vi "PH_HamamatsuCamera.ProcCases.vi"(0 "i ref in":refnum<vi>, 1 "selector":string, 2 "data":T1, 3 "call cluster":T2={"Object"="", "Selector"="", "CallType"=enum."synchronous", "Async Object"="", "Async Selector"="", "Data Descriptor"="", "Data"=[], "Error #"=0, "Expire"=0}, 5 "error in":errorcluster) -> (14 "i ref out":refnum<vi>, 17 "answer cluster":T2={"Object"="", "Selector"="", "CallType"=enum."synchronous", "Async Object"="", "Async Selector"="", "Data Descriptor"="", "Data"=[], "Error #"=0, "Expire"=0}, 19 "error out":errorcluster)   [LabVIEW 2014, in "PH_HamamatsuCamera.lvlib"]
doc: "This method is called by a process from within the default case in the event loop. The methods of a class that are linked to events will be called from THIS method. Add your code here."
uses:
  PH_HamamatsuCamera.lvlib
  CS_Core/CSSystem/CoreDefs/CoreDefs.call_type.ctl
  CS_Core/BaseProcess/BaseProcess.descriptor string definition.ctl
  CS_Core/CSSystem/CoreDefs/CoreDefs.rawDataType.ctl
  PH_HamamatsuCamera.Trigger Parameter.ctl
  PH_HamamatsuCamera.ROI.ctl
  CS_Core/CSSystem/CoreLib/CoreLib.string 2 byte array.vi
  CS_Core/CSSystem/CoreLib/CoreLib.byte array 2 double.vi
  CS_Core/CSSystem/CoreLib/CoreLib.byte array 2 string.vi
  CS_Core/CSSystem/CoreLib/CoreLib.byte array 2 int.vi
  CS_Core/CSSystem/CoreLib/CoreLib.lvlib
  CS_Core/BaseProcess/BaseProcess.lvlib
  CS_Core/CAEObj/CAEObj.lvlib
  PH_Basics/PH_PSDBWriter/PH_PSDBWriter.lvlib
  PH_Basics/PH_Cam_BaseClass/PH_Cam_BaseClass.lvlib
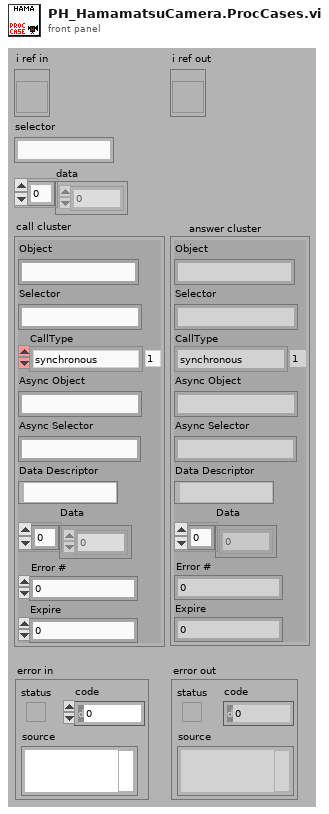
[diagram p1: front panel]
types:
  T1 = typedef "CoreDefs.rawDataType.ctl" = i8[]
  T2 = typedef "CoreDefs.call_type.ctl" = cluster{"Object":string, "Selector":string, "CallType":enum16{"simple", "synchronous", "asynchronous"}, "Async Object":string, "Async Selector":string, "Data Descriptor":T3, "Data":T1, "Error #":i32, "Expire":u32}
  T3 = typedef "BaseProcess.lvlib/BaseProcess.descriptor string definition.ctl" = string
  T4 = typedef "PH_HamamatsuCamera.lvlib/PH_HamamatsuCamera.Trigger Parameter.ctl" = cluster{"Mode":u32, "Polarity":u32, "Times":u32, "Delay":dbl}
  T5 = typedef "PH_HamamatsuCamera.lvlib/PH_HamamatsuCamera.ROI.ctl" = cluster{"Horizontal Offset":i32, "Vertical Offset":i32, "Horizontal Width":i32, "Vertical Width":i32}
  T6 = typedef "PH_PSDBWriter.lvlib/PH_PSDBWriter.PHELIX-Subsystems.ctl" = i32
  T7 = typedef "PH_HamamatsuCamera.lvlib/PH_HamamatsuCamera.i attribute.ctl" = cluster{"Gui Refs":cluster{"Camera Details":refnum<vi>, "ROI":refnum<vi>, "Set ROI to Maximum":refnum<vi>, "Trigger Parameters":refnum<vi>, "Brightness":refnum<vi>, "Shutter":refnum<vi>, "Gain":refnum<vi>, "Trigger Timeout":refnum<vi>, "Trigger Polarity":refnum<vi>, "Trigger Mode":refnum<vi>, "Parameters":refnum<vi>, "Set Cam Parameter":refnum<vi>, "Parameter to set":refnum<vi>, "Value to set":refnum<vi>}, "Cam":cluster{"Handle":i32, "Details":cluster{"Model":string, "Camera ID":string, "Firmware":string}, "Buffer Info":cluster{"height":u32, "width":u32, "datatype":u32}}, "H Offset":cluster{"Value":i32, "Minimum":i32, "Maximum":i32, "Increment":i32}, "V Offset":cluster{"Value":i32, "Minimum":i32, "Maximum":i32, "Increment":i32}, "H Width":cluster{"Value":i32, "Minimum":i32, "Maximum":i32, "Increment":i32}, "V Width":cluster{"Value":i32, "Minimum":i32, "Maximum":i32, "Increment":i32}, "Trigger Parameters":T4, "Trigger Timeout":u32, "Parameters":T8[], "Indicees Cam Parameters":cluster{"Brightness":i32, "Shutter":i32, "Gain":i32}, "Wanted Values":cluster{"Trigger Settings":T4[], "ROI":T5[], "Parameter":cluster{"Name":string, "Value":dbl}[]}}
  T8 = typedef "PH_HamamatsuCamera.lvlib/PH_HamamatsuCamera.Parameter Set.ctl" = cluster{"Parameter":string, "Value":dbl, "Writable":bool, "Range":cluster{"min":dbl, "max":dbl, "step":dbl}, "Default":dbl, "Value Names":cluster{"Name":string, "Value":dbl}[], "Text Values":bool}
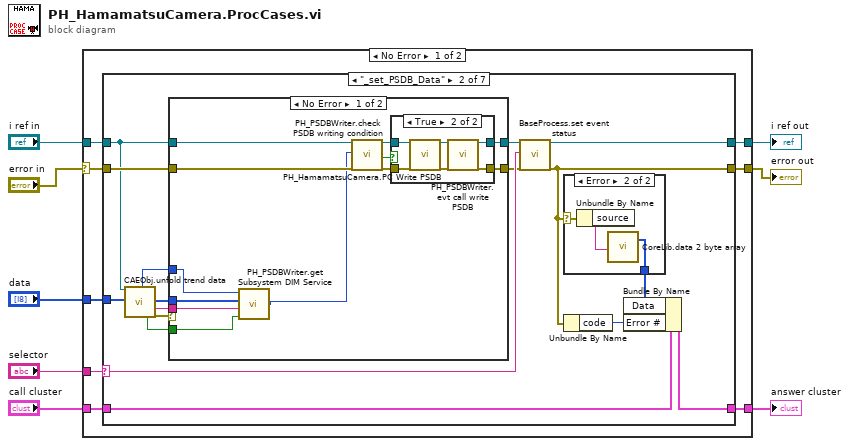
[diagram p0: block diagram]
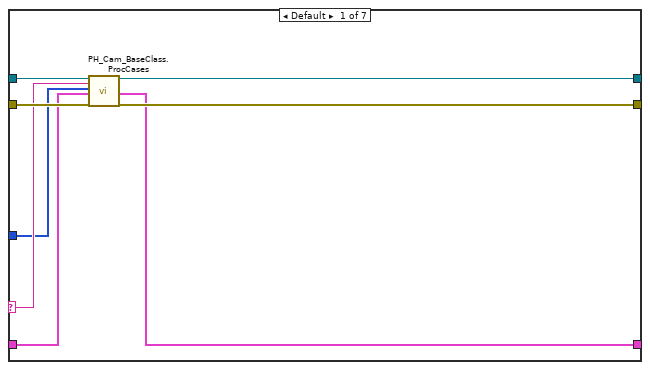
[diagram p2: hidden frame]
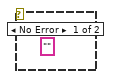
[diagram p5: hidden frame]
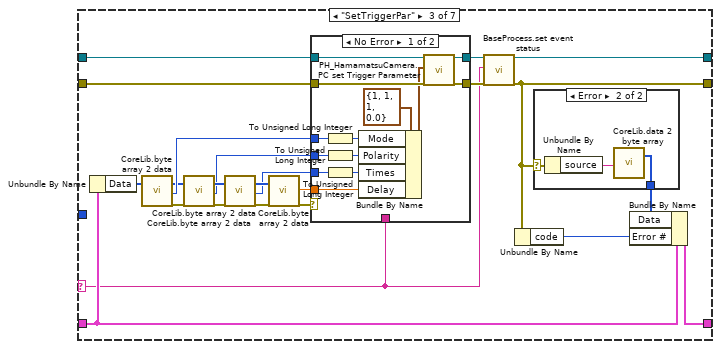
[diagram p6: hidden frame]
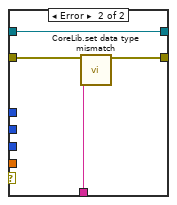
[diagram p8: hidden frame]
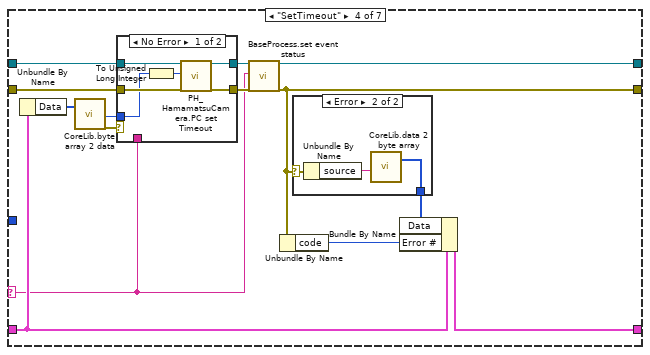
[diagram p9: hidden frame]
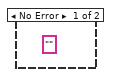
[diagram p10: hidden frame]
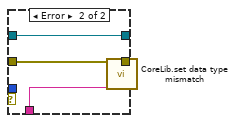
[diagram p11: hidden frame]
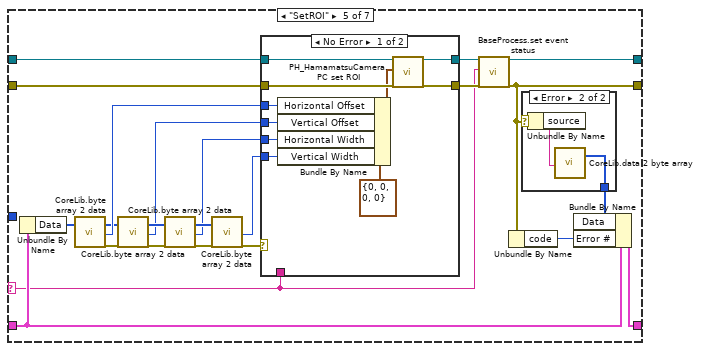
[diagram p12: hidden frame]
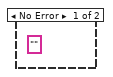
[diagram p13: hidden frame]
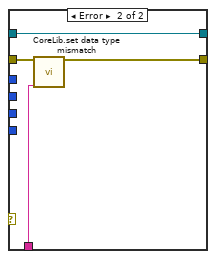
[diagram p14: hidden frame]
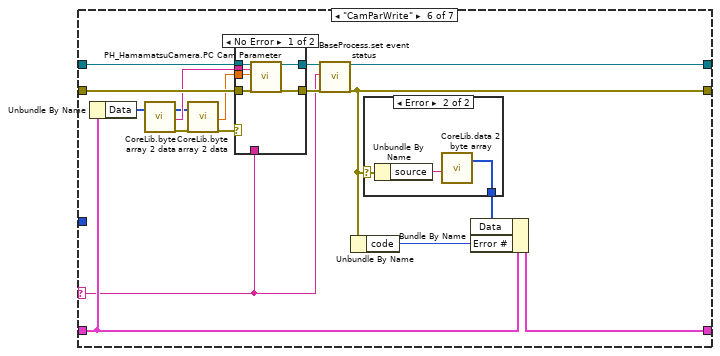
[diagram p15: hidden frame]
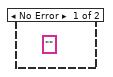
[diagram p16: hidden frame]
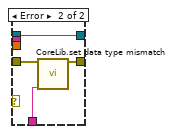
[diagram p17: hidden frame]
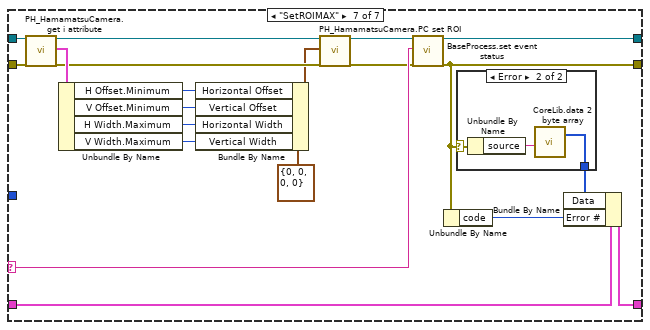
[diagram p18: hidden frame]
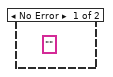
[diagram p19: hidden frame]
diagram:
  n1 = case shown="No Error" "error in" {
    selector: "error in" -> [w9 w231]
    tunnel: "selector" -> [w16 _]
    tunnel: [w15 w230] -> w7
    tunnel: "call cluster" -> [w14 w230]
    tunnel: "i ref in" -> [w13 w232]
    tunnel: [w12 w232] -> w4
    tunnel: [w11 w231] -> w3
    tunnel: "data" -> [w10 _]
    frame No Error {
      n2 = case shown="\"_set_PSDB_Data\"" w16 {
        selector: w16 -> [w19 w37 w81 w115 w151 w185 w220]
        tunnel: w13 -> [w18 w28 w89 w123 w159 w193 w226]
        tunnel: [w24 w36 w80 w114 w150 w184 w219] -> w12
        tunnel: w14 -> [w20 w40 w86 w120 w156 w190 w223]
        tunnel: [w21 w39 w85 w119 w155 w189 w222] -> w15
        tunnel: w9 -> [w23 w29 w88 w122 w158 w192 w225]
        tunnel: [w22 w38 w82 w116 w152 w186 w221] -> w11
        tunnel: w10 -> [w17 w25 _ _ _ _ _]
        frame Default {
          # "In the default case, always call the ProcCase method of the parent class"
          n3 = call "PH_Cam_BaseClass.ProcCases.vi"("i ref in"=w18, "selector"=w19, "data"=w17, "call cluster"=w20, "error in"=w23) -> ("i ref out"=w24:refnum<vi>, "answer cluster"=w21:T2, "error out"=w22:errorcluster)  [unwired: 12 in]
        }
        frame "_set_PSDB_Data" {
          n4 = call "CAEObj.unfold trend data.vi"("i ref in"=w28, "raw trend data"=w25) -> ("quality"=w30:i32, "no link"=w33:bool, "data"=w31:i8[], "typeDescriptor"=w32:string, "error out"=w34:errorcluster)  [unwired: 9 in, 4 out]
          n5 = case shown="No Error" w34 {
            tunnel: w29 -> [w53 w63]
            tunnel: [w52 w62] -> w27
            tunnel: [w51 w63] -> w26
            tunnel: w28 -> [w49 w62]
            tunnel: w33 -> [w43 _]
            tunnel: w32 -> [w44 _]
            tunnel: w31 -> [w46 _]
            tunnel: w30 -> [w45 _]
            frame No Error {
              n6 = call "PH_PSDBWriter.get Subsystem DIM Service.vi"("no link"=w43, "typeDescriptor"=w44, "data"=w46, "quality"=w45) -> ("PHELIX Subsystems"=w42:T6)
              n7 = call "PH_PSDBWriter.check PSDB writing condition.vi"("i ref in"=w49, "wanted Subsystem"=w42, "error IO"=w53) -> ("i ref out"=w48:refnum<vi>, "write PSDB?"=w47:bool, "error out"=w50:errorcluster)  [unwired: 14 in]
              n8 = case shown="True" w47 {
                tunnel: w50 -> [w54 w61]
                tunnel: [w55 w58] -> w52
                tunnel: [w54 w56] -> w51
                tunnel: w48 -> [w55 w60]
                frame False {
                }
                frame True {
                  n9 = call "PH_HamamatsuCamera.PC Write PSDB.vi"("i ref in"=w60, "error IO"=w61) -> ("i ref out"=w59:refnum<vi>, "error out"=w57:errorcluster)  [unwired: 16 in]
                  n10 = call "PH_PSDBWriter.evt call write PSDB.vi"("i ref in"=w59, "error in (no error)"=w57) -> ("i ref out"=w58:refnum<vi>, "error out"=w56:errorcluster)  [unwired: 16 in]
                }
              }
            }
            frame Error {
            }
          }
          n11 = call "BaseProcess.set event status.vi"("i ref in"=w27, "EventStatus"=w37, "error in (no error)"=w26) -> ("i ref out"=w36:refnum<vi>, "error out"=w38:errorcluster)  [unwired: 14 in, 1 out]
          n12 = case shown="Error" w38 {
            selector: w38 -> [_ w66]
            tunnel: [_ w64] -> w35
            frame No Error {
              (unwired) "" ("source")
            }
            frame Error {
              n13 = Unbundle By Name(w66) -> ("source"=w65:string)
              n14 = call-poly "CoreLib.data 2 byte array.vi"("string"=w65) -> ("byteArray out"=w64:T1)  [unwired: 18 in]
            }
          }
          n15 = Unbundle By Name(w38) -> ("code"=w41:i32)
          n16 = Bundle By Name(cluster=w40, "Data"=w35, "Error #"=w41) -> (w39:T2)
        }
        frame "SetTriggerPar" {
          n17 = Unbundle By Name(w86) -> ("Data"=w79:T1)
          n18 = call-poly "CoreLib.byte array 2 data.vi"("byteArray"=w79) -> ("byteArray out"=w72:T1, "i32"=w73:i32, "error out"=w77:errorcluster)  [unwired: 16 in]
          n19 = call-poly "CoreLib.byte array 2 data.vi"("byteArray"=w72, "error in (no error)"=w77) -> ("byteArray out"=w71:T1, "i32"=w69:i32, "error out"=w75:errorcluster)  [unwired: 15 in]
          n20 = call-poly "CoreLib.byte array 2 data.vi"("byteArray"=w71, "error in (no error)"=w75) -> ("byteArray out"=w70:T1, "i32"=w68:i32, "error out"=w76:errorcluster)  [unwired: 15 in]
          n21 = call-poly "CoreLib.byte array 2 data.vi"("byteArray"=w70, "error in (no error)"=w76) -> ("d64"=w67:dbl, "error out"=w74:errorcluster)  [unwired: 15 in, 1 out]
          n22 = case shown="No Error" w74 {
            tunnel: [w94 w109] -> w84
            tunnel: w89 -> [w104 w109]
            tunnel: w88 -> [w105 w108]
            tunnel: [w93 w107] -> w83
            tunnel: w81 -> [_ w106]
            tunnel: w73 -> [w101 _]
            tunnel: w69 -> [w99 _]
            tunnel: w68 -> [w98 _]
            tunnel: w67 -> [w97 _]
            frame No Error {
              n23 = To Unsigned Long Integer(number=w101) -> (unsigned 32bit integer=w100:u32)
              n24 = To Unsigned Long Integer(number=w99) -> (unsigned 32bit integer=w96:u32)
              n25 = To Unsigned Long Integer(number=w98) -> (unsigned 32bit integer=w95:u32)
              n26 = Bundle By Name(cluster=T4 {"Mode"=1, "Polarity"=1, "Times"=1, "Delay"=0.0} ("Trigger Parameters"), "Mode"=w100, "Polarity"=w96, "Times"=w95, "Delay"=w97) -> (w102:T4)
              n27 = call "PH_HamamatsuCamera.PC set Trigger Parameter.vi"("i ref in"=w104, "Trigger Parameters"=w102, "error in (no error)"=w105) -> ("i ref out"=w94:refnum<vi>, "error out"=w93:errorcluster)  [unwired: 15 in]
            }
            frame Error {
              n28 = call "CoreLib.set data type mismatch.vi"("error in (no error)"=w108, "error source"=w106) -> ("error out"=w107:errorcluster)  [unwired: 17 in]
            }
          }
          n29 = call "BaseProcess.set event status.vi"("i ref in"=w84, "EventStatus"=w81, "error in (no error)"=w83) -> ("i ref out"=w80:refnum<vi>, "error out"=w82:errorcluster)  [unwired: 14 in, 1 out]
          n30 = Unbundle By Name(w82) -> ("code"=w87:i32)
          n31 = case shown="Error" w82 {
            selector: w82 -> [_ w92]
            tunnel: [_ w91] -> w78
            frame No Error {
            }
            frame Error {
              n32 = Unbundle By Name(w92) -> ("source"=w90:string)
              n33 = call-poly "CoreLib.data 2 byte array.vi"("string"=w90) -> ("byteArray out"=w91:T1)  [unwired: 18 in]
            }
          }
          n34 = Bundle By Name(cluster=w86, "Data"=w78, "Error #"=w87) -> (w85:T2)
        }
        frame "SetTimeout" {
          n35 = Unbundle By Name(w120) -> ("Data"=w113:T1)
          n36 = call-poly "CoreLib.byte array 2 data.vi"("byteArray"=w113) -> ("i32"=w112:i32, "error out"=w111:errorcluster)  [unwired: 16 in, 1 out]
          n37 = case shown="No Error" w111 {
            tunnel: [w128 w136] -> w118
            tunnel: w123 -> [w131 w136]
            tunnel: w122 -> [w132 w135]
            tunnel: [w127 w134] -> w117
            tunnel: w115 -> [_ w133]
            tunnel: w112 -> [w130 _]
            frame No Error {
              n38 = To Unsigned Long Integer(number=w130) -> (unsigned 32bit integer=w129:u32)
              n39 = call "PH_HamamatsuCamera.PC set Timeout.vi"("i ref in"=w131, "Timeout"=w129, "error in (no error)"=w132) -> ("i ref out"=w128:refnum<vi>, "error out"=w127:errorcluster)  [unwired: 15 in]
            }
            frame Error {
              n40 = call "CoreLib.set data type mismatch.vi"("error in (no error)"=w135, "error source"=w133) -> ("error out"=w134:errorcluster)  [unwired: 17 in]
            }
          }
          n41 = call "BaseProcess.set event status.vi"("i ref in"=w118, "EventStatus"=w115, "error in (no error)"=w117) -> ("i ref out"=w114:refnum<vi>, "error out"=w116:errorcluster)  [unwired: 14 in, 1 out]
          n42 = Unbundle By Name(w116) -> ("code"=w121:i32)
          n43 = case shown="Error" w116 {
            selector: w116 -> [_ w126]
            tunnel: [_ w124] -> w110
            frame No Error {
              (unwired) "" ("source")
            }
            frame Error {
              n44 = Unbundle By Name(w126) -> ("source"=w125:string)
              n45 = call-poly "CoreLib.data 2 byte array.vi"("string"=w125) -> ("byteArray out"=w124:T1)  [unwired: 18 in]
            }
          }
          n46 = Bundle By Name(cluster=w120, "Data"=w110, "Error #"=w121) -> (w119:T2)
        }
        frame "SetROI" {
          n47 = Unbundle By Name(w156) -> ("Data"=w149:T1)
          n48 = call-poly "CoreLib.byte array 2 data.vi"("byteArray"=w149) -> ("byteArray out"=w142:T1, "i32"=w148:i32, "error out"=w144:errorcluster)  [unwired: 16 in]
          n49 = call-poly "CoreLib.byte array 2 data.vi"("byteArray"=w142, "error in (no error)"=w144) -> ("byteArray out"=w141:T1, "i32"=w139:i32, "error out"=w146:errorcluster)  [unwired: 15 in]
          n50 = call-poly "CoreLib.byte array 2 data.vi"("byteArray"=w141, "error in (no error)"=w146) -> ("byteArray out"=w140:T1, "i32"=w138:i32, "error out"=w145:errorcluster)  [unwired: 15 in]
          n51 = call-poly "CoreLib.byte array 2 data.vi"("byteArray"=w140, "error in (no error)"=w145) -> ("i32"=w137:i32, "error out"=w143:errorcluster)  [unwired: 15 in, 1 out]
          n52 = case shown="No Error" w143 {
            tunnel: [w170 w176] -> w154
            tunnel: w159 -> [w171 w176]
            tunnel: w158 -> [w172 w175]
            tunnel: [w169 w174] -> w153
            tunnel: w151 -> [_ w173]
            tunnel: w148 -> [w167 _]
            tunnel: w139 -> [w166 _]
            tunnel: w138 -> [w164 _]
            tunnel: w137 -> [w165 _]
            frame No Error {
              n53 = Bundle By Name(cluster=T5 {"Horizontal Offset"=0, "Vertical Offset"=0, "Horizontal Width"=0, "Vertical Width"=0} ("ROI"), "Horizontal Offset"=w167, "Vertical Offset"=w166, "Horizontal Width"=w164, "Vertical Width"=w165) -> (w163:T5)
              n54 = call "PH_HamamatsuCamera.PC set ROI.vi"("VI in"=w171, "Horizontal Offset"=w163, "error in (no error)"=w172) -> ("VI out"=w170:refnum<vi>, "error out"=w169:errorcluster)  [unwired: 15 in]
            }
            frame Error {
              n55 = call "CoreLib.set data type mismatch.vi"("error in (no error)"=w175, "error source"=w173) -> ("error out"=w174:errorcluster)  [unwired: 17 in]
            }
          }
          n56 = call "BaseProcess.set event status.vi"("i ref in"=w154, "EventStatus"=w151, "error in (no error)"=w153) -> ("i ref out"=w150:refnum<vi>, "error out"=w152:errorcluster)  [unwired: 14 in, 1 out]
          n57 = Unbundle By Name(w152) -> ("code"=w157:i32)
          n58 = case shown="Error" w152 {
            selector: w152 -> [_ w162]
            tunnel: [_ w160] -> w147
            frame No Error {
              (unwired) "" ("source")
            }
            frame Error {
              n59 = Unbundle By Name(w162) -> ("source"=w161:string)
              n60 = call-poly "CoreLib.data 2 byte array.vi"("string"=w161) -> ("byteArray out"=w160:T1)  [unwired: 18 in]
            }
          }
          n61 = Bundle By Name(cluster=w156, "Data"=w147, "Error #"=w157) -> (w155:T2)
        }
        frame "CamParWrite" {
          n62 = Unbundle By Name(w190) -> ("Data"=w183:T1)
          n63 = call-poly "CoreLib.byte array 2 data.vi"("byteArray"=w183) -> ("byteArray out"=w179:T1, "string"=w182:string, "error out"=w180:errorcluster)  [unwired: 16 in]
          n64 = call-poly "CoreLib.byte array 2 data.vi"("byteArray"=w179, "error in (no error)"=w180) -> ("d64"=w178:dbl, "error out"=w177:errorcluster)  [unwired: 15 in, 1 out]
          n65 = case shown="No Error" w177 {
            tunnel: [w198 w206] -> w188
            tunnel: w193 -> [w201 w206]
            tunnel: w192 -> [w202 w205]
            tunnel: [w197 w204] -> w187
            tunnel: w185 -> [_ w203]
            tunnel: w182 -> [w199 _]
            tunnel: w178 -> [w200 _]
            frame No Error {
              n66 = call "PH_HamamatsuCamera.PC Cam Parameter.vi"("VI in"=w201, "Parameter Name"=w199, "Wanted Value"=w200, "error in (no error)"=w202) -> ("VI out"=w198:refnum<vi>, "error out"=w197:errorcluster)  [unwired: 14 in]
            }
            frame Error {
              n67 = call "CoreLib.set data type mismatch.vi"("error in (no error)"=w205, "error source"=w203) -> ("error out"=w204:errorcluster)  [unwired: 17 in]
            }
          }
          n68 = call "BaseProcess.set event status.vi"("i ref in"=w188, "EventStatus"=w185, "error in (no error)"=w187) -> ("i ref out"=w184:refnum<vi>, "error out"=w186:errorcluster)  [unwired: 14 in, 1 out]
          n69 = Unbundle By Name(w186) -> ("code"=w191:i32)
          n70 = case shown="Error" w186 {
            selector: w186 -> [_ w196]
            tunnel: [_ w194] -> w181
            frame No Error {
              (unwired) "" ("source")
            }
            frame Error {
              n71 = Unbundle By Name(w196) -> ("source"=w195:string)
              n72 = call-poly "CoreLib.data 2 byte array.vi"("string"=w195) -> ("byteArray out"=w194:T1)  [unwired: 18 in]
            }
          }
          n73 = Bundle By Name(cluster=w190, "Data"=w181, "Error #"=w191) -> (w189:T2)
        }
        frame "SetROIMAX" {
          n74 = call "PH_HamamatsuCamera.get i attribute.vi"("i ref in"=w226, "error in (no error)"=w225) -> ("i ref out"=w216:refnum<vi>, "i attribute"=w217:T7, "error out"=w215:errorcluster)  [unwired: 15 in]
          n75 = Unbundle By Name(w217) -> ("H Offset.Minimum"=w211:i32, "V Offset.Minimum"=w209:i32, "H Width.Maximum"=w208:i32, "V Width.Maximum"=w207:i32)
          n76 = Bundle By Name(cluster=T5 {"Horizontal Offset"=0, "Vertical Offset"=0, "Horizontal Width"=0, "Vertical Width"=0} ("ROI"), "Horizontal Offset"=w211, "Vertical Offset"=w209, "Horizontal Width"=w208, "Vertical Width"=w207) -> (w210:T5)
          n77 = call "PH_HamamatsuCamera.PC set ROI.vi"("VI in"=w216, "Horizontal Offset"=w210, "error in (no error)"=w215) -> ("VI out"=w214:refnum<vi>, "error out"=w213:errorcluster)  [unwired: 15 in]
          n78 = call "BaseProcess.set event status.vi"("i ref in"=w214, "EventStatus"=w220, "error in (no error)"=w213) -> ("i ref out"=w219:refnum<vi>, "error out"=w221:errorcluster)  [unwired: 14 in, 1 out]
          n79 = Unbundle By Name(w221) -> ("code"=w224:i32)
          n80 = case shown="Error" w221 {
            selector: w221 -> [_ w229]
            tunnel: [_ w227] -> w218
            frame No Error {
              (unwired) "" ("source")
            }
            frame Error {
              n81 = Unbundle By Name(w229) -> ("source"=w228:string)
              n82 = call-poly "CoreLib.data 2 byte array.vi"("string"=w228) -> ("byteArray out"=w227:T1)  [unwired: 18 in]
            }
          }
          n83 = Bundle By Name(cluster=w223, "Data"=w218, "Error #"=w224) -> (w222:T2)
        }
      }
    }
    frame Error {
    }
  }
  "answer cluster" <- w7
  "i ref out" <- w4
  "error out" <- w3
